vi "delete operation by line.vi"(8 "error in":errorcluster, 10 "line to delete":T1, 11 "Scan Engine editor node in":refnum<class "Scan Engine editor node.lvclass">) -> (0 "error out":errorcluster, 3 "Scan Engine editor node out":refnum<class "Scan Engine editor node.lvclass">)   [LabVIEW 2013, in "Scan Engine editor node.lvclass"]
uses:
  Scan Engine editor node.lvclass
  table line.ctl
  <vilib>/NI/Tag Bus Module Framework/channel/TBM channel.lvclass
  read actual configuration.vi
  write actual configuration.vi
  <vilib>/NI/TBM Modules/variable/module/configuration/Scan Engine configuration.lvclass
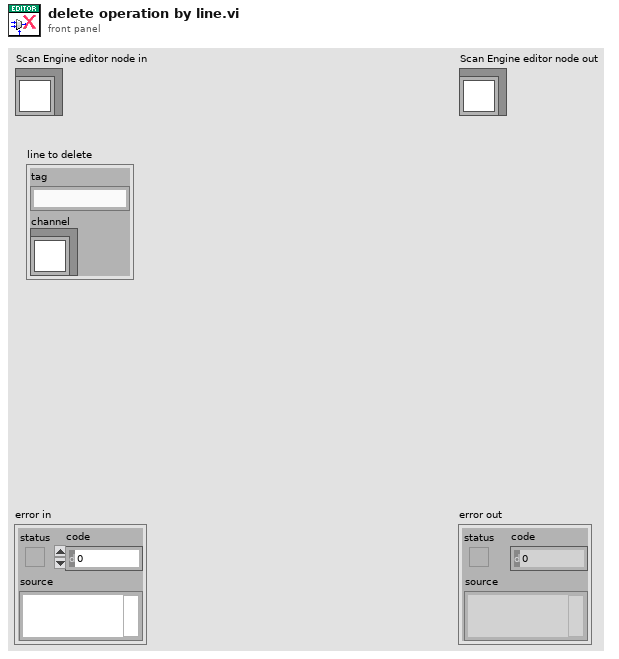
[diagram p1: front panel]
types:
  T1 = typedef "Scan Engine editor node.lvclass/table line.ctl" = cluster{"tag":string, "channel":refnum<class "TBM channel.lvclass">}
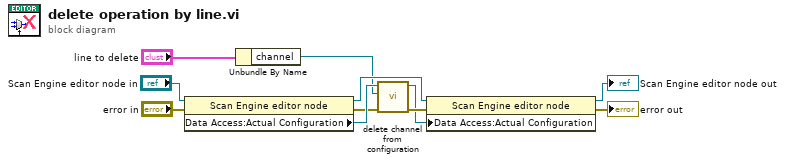
[diagram p0: block diagram]
diagram:
  n1 = property class="Scan Engine editor node"(reference="Scan Engine editor node in", error in="error in") -> (reference out=w8:refnum<class "Scan Engine editor node.lvclass">, error out=w4:errorcluster, "Data Access:Actual Configuration"=w5:refnum<class "Scan Engine configuration.lvclass">)
  n2 = Unbundle By Name("line to delete") -> ("channel"=w1:refnum<class "TBM channel.lvclass">)
  n3 = call <vilib>:"delete channel from configuration.vi"("error in"=w4, "channel"=w1, "Scan Engine configuration in"=w5) -> ("error out"=w3:errorcluster, "Scan Engine configuration out"=w2:refnum<class "Scan Engine configuration.lvclass">)  [unwired: 7 in]
  n4 = property class="Scan Engine editor node"(reference=w8, error in=w3, "Data Access:Actual Configuration"=w2) -> (reference out=→"Scan Engine editor node out":refnum<class "Scan Engine editor node.lvclass">, error out=→"error out":errorcluster)
